vi "Configure Calibration Kit.vi"(7 "Connector type":T1(ring), 8 "error in (no error)":errorcluster, 10 "Cal kit Name":string, 11 "VNA-ENA in":refnum<class "VNA-ENA.lvclass">) -> (0 "error out":errorcluster, 3 "VNA-ENA out":refnum<class "VNA-ENA.lvclass">)   [LabVIEW 2020, in "VNA-ENA.lvclass"]
doc: "Configure the calibration kit to use."
uses:
  VNA-ENA.lvclass
  C:/Sandbox/Git_Sandbox/WiSpry Test Framework source code (LV20)/WiSpry Test Framework/Instruments/Instrument.lvclass
  Instrument.lvclass
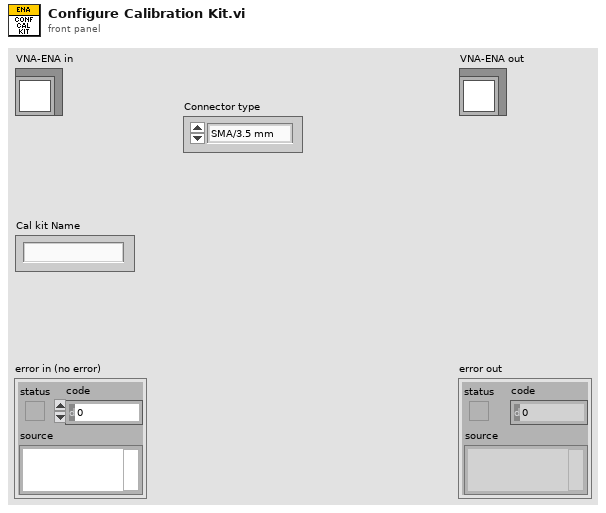
[diagram p1: front panel]
types:
  T1 = enum16{"SMA/3.5 mm", "2.92 mm", "2.4 mm", "1.85 mm", "N 50 Ohm", "N 75 Ohm", "7-16"}
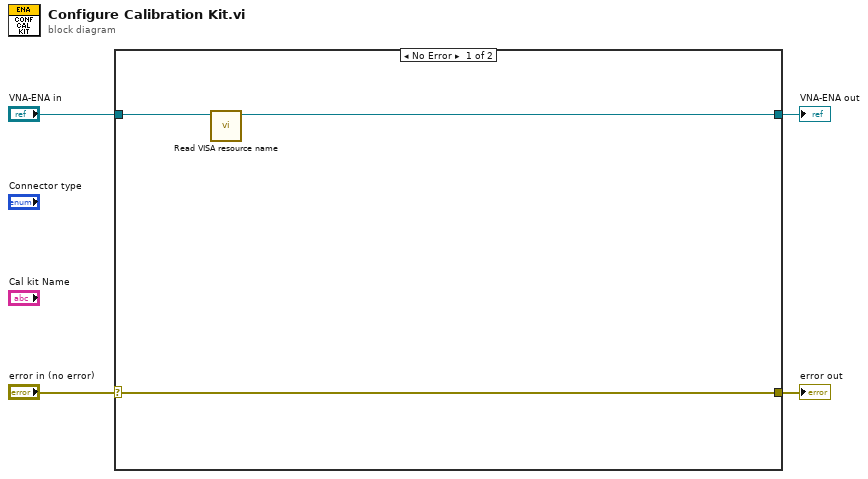
[diagram p0: block diagram]
diagram:
  n1 = case shown="No Error" "error in (no error)" {
    selector: "error in (no error)" -> [w5 w9]
    tunnel: [w5 w9] -> w4
    tunnel: [w6 w8] -> w3
    tunnel: "VNA-ENA in" -> [w7 w8]
    frame No Error {
      n2 = call "Read VISA resource name.vi"("Instrument in"=w7) -> ("Instrument out"=w6:refnum<class "VNA-ENA.lvclass">)  [unwired: 9 in, 1 out]
    }
    frame Error {
    }
  }
  "error out" <- w4
  "VNA-ENA out" <- w3
